vi "AccumulatingDifferences.vi"(6 "Reset":bool, 11 "input":i16) -> (3 "Accumulator":u64)   [LabVIEW 2014]
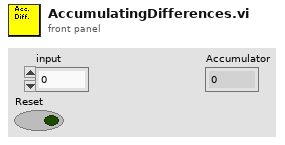
[diagram p1: front panel]
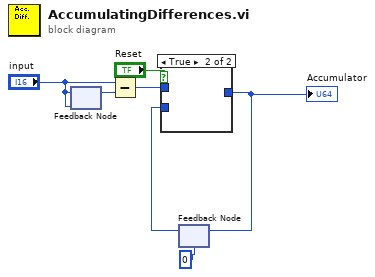
[diagram p0: block diagram]
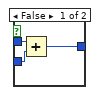
[diagram p2: hidden frame]
diagram:
  n1 = feedback #1("input") -> (w5:i16)
  n2 = feedback-in #1("input") -> ()
  n3 = Subtract(x="input", y=w5) -> (x-y=w4:i16)
  n4 = feedback #2(u64 0) -> (w3:u64)
  n5 = case shown="True" "Reset" {
    tunnel: [w10 _] -> w6
    tunnel: w4 -> [w9 _]
    tunnel: w3 -> [w8 _]
    frame False {
      n6 = Add(x=w9, y=w8) -> (x+y=w10:u64)
    }
    frame True {
    }
  }
  "Accumulator" <- w6
  n7 = feedback-in #2(w6) -> ()
